vi "UT_FX5U_SLMP.vi"() -> ()   [LabVIEW 2019]
uses:
  FX5U SLMP Binary/FX5U SLMP Binary.lvlib
panel:
  in  "IP:Port":string="192.168.3.70:1234"
  out "Success":bool
  out "Error":bool
  in  "Close API":bool
  out "TCP connected":bool
  in  "D Array":i16[](array[numeric])=[0, -30, 0, 50, 79, 69, 90, 0, 0, 80, 0, 0]
  in  "Wr D Length (U16)":u16=10
  in  "Wr D Position (U32)":u32=7500
  in  "Write Multi-D":bool
  in  "Wr M Length (U16)":u16=10
  in  "Wr M Start Position (U32)":u32=6500
  in  "M Data input":bool[](array[boolean])=[FALSE, FALSE, TRUE, FALSE, FALSE, TRUE, FALSE, FALSE, FALSE, TRUE, FALSE, FALSE, FALSE, FALSE, TRUE, TRUE]
  in  "Write Multi-M":bool
  in  "Rd D Length (U16)":u16=12
  in  "Rd D Start Position (U32)":u32=7500
  in  "Write Unit-D":bool
  in  "Read Multi-D":bool
  out "Error Out":errorcluster
  in  "Error In":errorcluster
  out "D Data out":i16[](array[numeric])=[0, 0, -12288, 0, -1, 3, 2, 0, 208, -256, 1023, 6656]
  out "M  Data out":bool[](array[boolean])=[FALSE, FALSE, FALSE, FALSE, FALSE, FALSE, FALSE, FALSE, FALSE, FALSE, FALSE, FALSE, FALSE, FALSE, TRUE, FALSE, FALSE, TRUE, FALSE, FALSE]
  in  "Wr D Position (U32)":u32=7500
  in  "D Data In":i16=50
  in  "M Data In":bool
  in  "Wr M Position (U32)":u32
  in  "Rd M Length (U16)":u16=20
  in  "Rd M Start Position (U32)":u32=6500
  in  "stop":bool
  in  "Read Multi-M":bool
  in  "Write Unit-M":bool
  in  "Connect PLC":bool
  # "傳輸格式: BINARY\n參考FX5U SLMP手冊編輯通訊架構\n已測試: FX5U 64M型號"
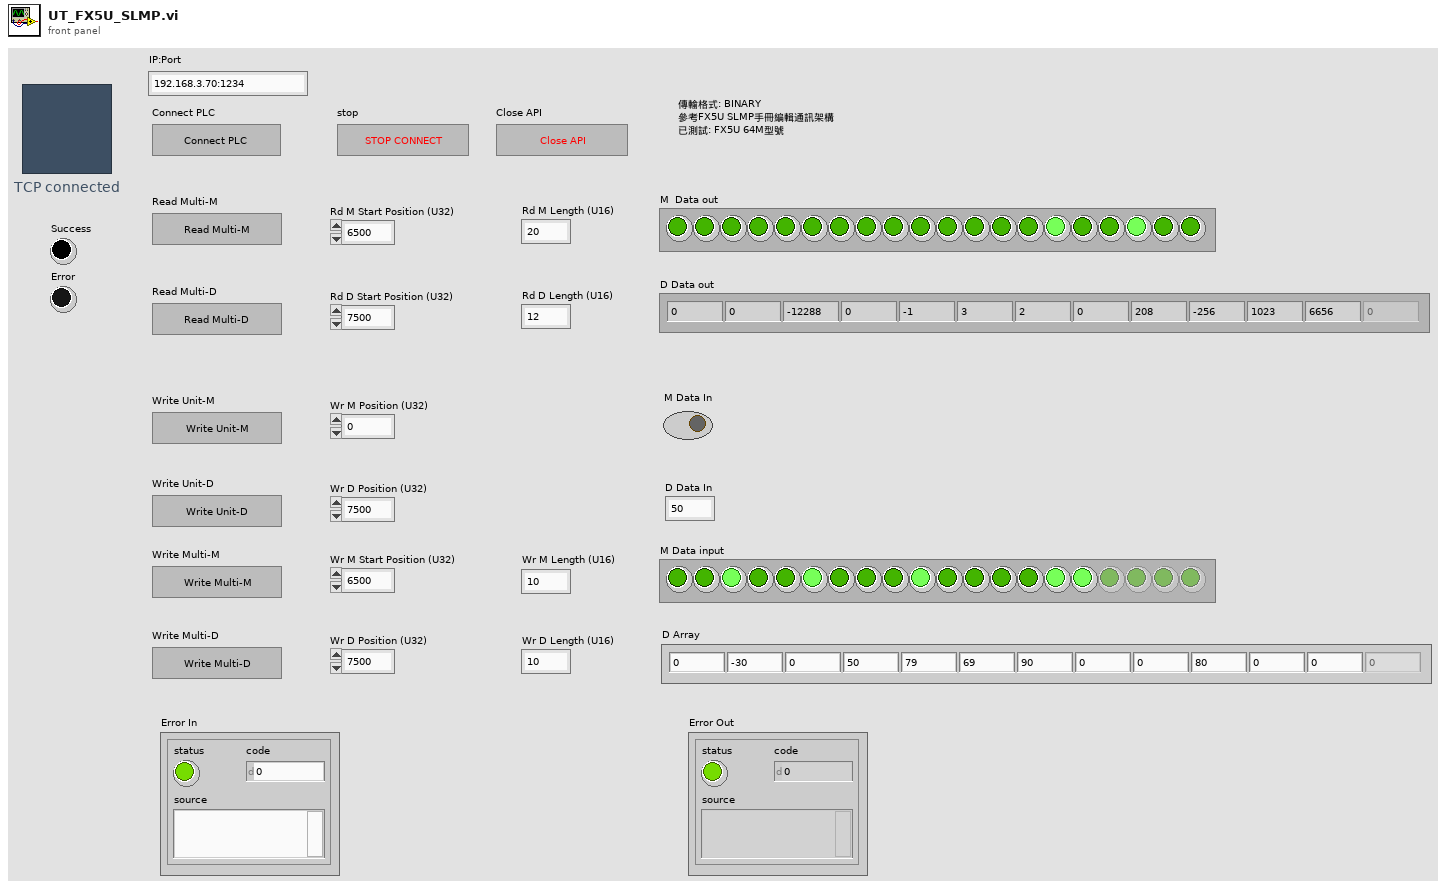
[diagram p1: front panel]
types:
  T1 = typedef "FX5U SLMP Binary.lvlib/Data Cluster.ctl" = cluster{"M Array":bool[], "D Array":i16[]}
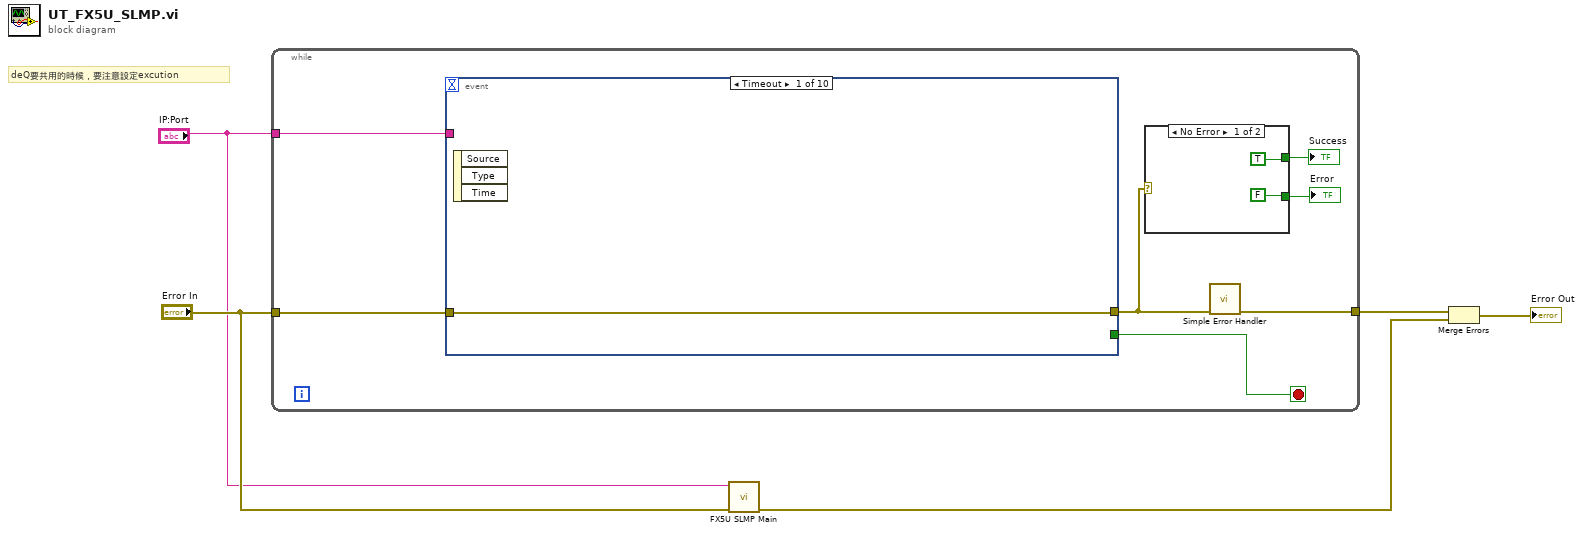
[diagram p0: block diagram]
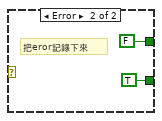
[diagram p2: hidden frame]
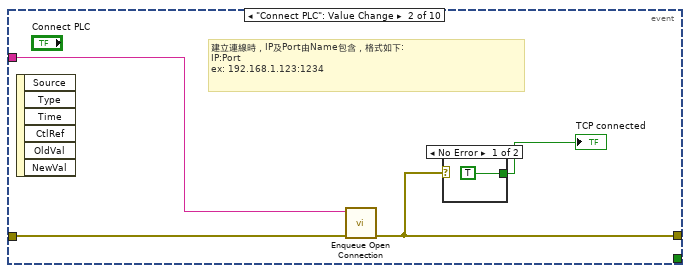
[diagram p3: hidden frame]
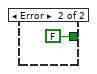
[diagram p4: hidden frame]
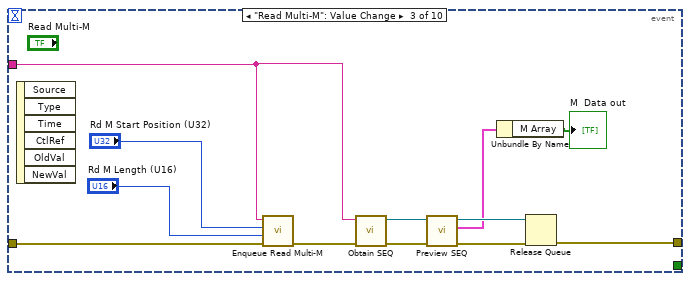
[diagram p5: hidden frame]
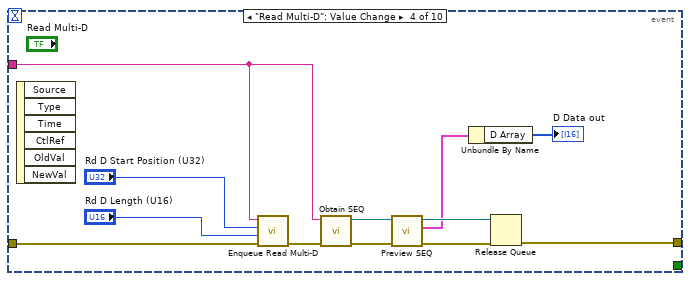
[diagram p6: hidden frame]
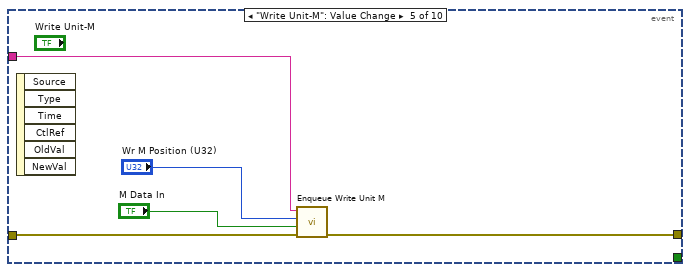
[diagram p7: hidden frame]
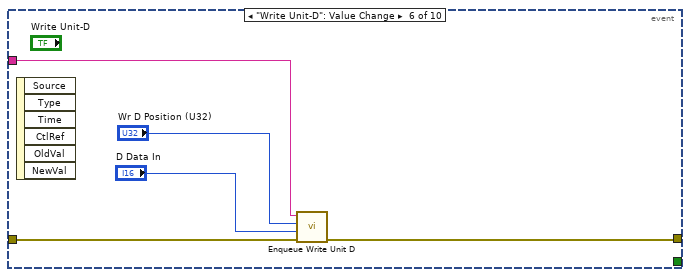
[diagram p8: hidden frame]
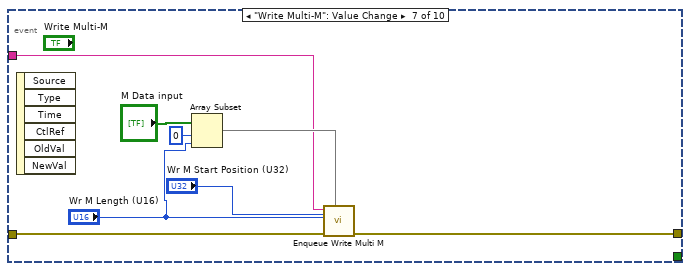
[diagram p9: hidden frame]
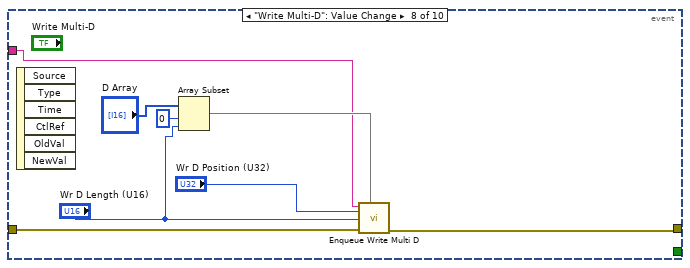
[diagram p10: hidden frame]
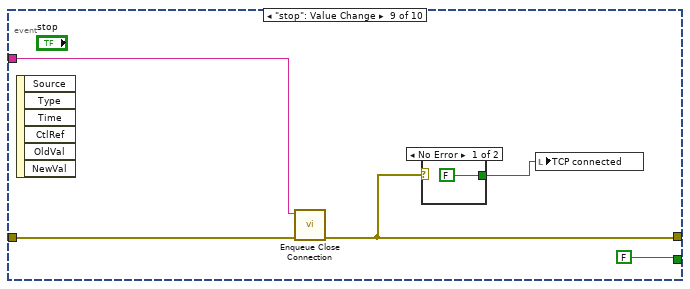
[diagram p11: hidden frame]
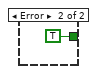
[diagram p12: hidden frame]
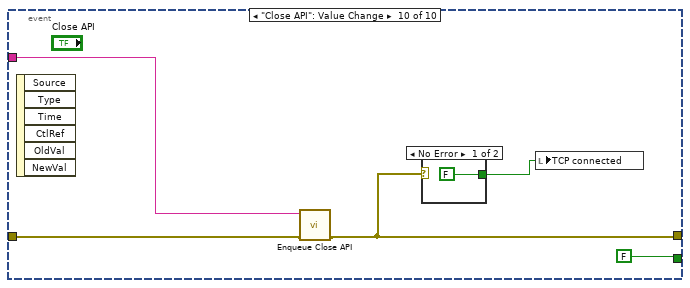
[diagram p13: hidden frame]
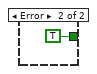
[diagram p14: hidden frame]
diagram:
  # "deQ要共用的時候，要注意設定excution"
  n1 = while {
    tunnel: "Error In" -> [w12]
    tunnel: [w11] -> w5
    tunnel: "IP:Port" -> [w6]
    stop <- w10 stop-if-true
    n2 = event shown="[0] Timeout" {
      selector: _ -> [_ _ _ _ _ _ _ _ _ _]
      dyn-events: _ -> [_ _ _ _ _ _ _ _ _ _]
      timeout: _ -> [_ _ _ _ _ _ _ _ _ _]
      tunnel: w12 -> [w17 w21 w35 w39 w50 w57 w64 w73 w78 w83]
      tunnel: [w17 w20 w31 w43 w49 w56 w63 w72 w76 w82] -> w7
      tunnel: [_ _ _ _ _ _ _ _ FALSE FALSE] -> w10
      tunnel: w6 -> [_ w18 w24 w36 w48 w53 w58 w66 w74 w81]
      event Timeout {
        n3 = event-data() -> ()  [unwired: 1 in, 3 out]
      }
      event "Connect PLC": Value Change {
        # "建立連線時，IP及Port由Name包含，格式如下:\nIP:Port\nex: 192.168.1.123:1234"
        n4 = event-data() -> ()  [unwired: 1 in, 6 out]
        n5 = call "Enqueue Open Connection.vi"("Error In"=w21, "Name"=w18) -> ("Error Out"=w20:errorcluster)  [unwired: 9 in]
        n6 = case shown="No Error" w20 {
          tunnel: [TRUE ("TCP connected") FALSE ("TCP connected")] -> w19
          frame No Error {
          }
          frame Error {
          }
        }
        "TCP connected" <- w19
      }
      event "Read Multi-M": Value Change {
        n7 = event-data() -> ()  [unwired: 1 in, 6 out]
        n8 = call "Enqueue Read Multi-M.vi"("Error In"=w35, "Length (U16)"="Rd M Length (U16)", "Start Position (U32)"="Rd M Start Position (U32)", "Name"=w24) -> ("Error Out"=w32:errorcluster)  [unwired: 7 in]
        n9 = call "Obtain SEQ.vi"("Error In"=w32, "Name"=w24) -> ("Error Out"=w30:errorcluster, "SEQ out"=w28:refnum<queue>)  [unwired: 8 in]
        n10 = call "Preview SEQ.vi"("Error In"=w30, "SEQ in"=w28) -> ("Error Out"=w29:errorcluster, "Data Cluster"=w26:T1, "SEQ out"=w27:refnum<queue>)  [unwired: 7 in]
        n11 = Unbundle By Name(w26) -> ("M Array"=→"M  Data out":bool[])
        n12 = Release Queue(queue=w27, error in (no error)=w29) -> (error out=w31:errorcluster)  [unwired: 1 in, 2 out]
      }
      event "Read Multi-D": Value Change {
        n13 = event-data() -> ()  [unwired: 1 in, 6 out]
        n14 = call "Enqueue Read Multi-D.vi"("Error In"=w39, "Length (U16)"="Rd D Length (U16)", "Start Position (U32)"="Rd D Start Position (U32)", "Name"=w36) -> ("Error Out"=w42:errorcluster)  [unwired: 7 in]
        n15 = call "Obtain SEQ.vi"("Error In"=w42, "Name"=w36) -> ("Error Out"=w47:errorcluster, "SEQ out"=w45:refnum<queue>)  [unwired: 8 in]
        n16 = call "Preview SEQ.vi"("Error In"=w47, "SEQ in"=w45) -> ("Error Out"=w46:errorcluster, "Data Cluster"=w38:T1, "SEQ out"=w44:refnum<queue>)  [unwired: 7 in]
        n17 = Unbundle By Name(w38) -> ("D Array"=→"D Data out":i16[])
        n18 = Release Queue(queue=w44, error in (no error)=w46) -> (error out=w43:errorcluster)  [unwired: 1 in, 2 out]
      }
      event "Write Unit-M": Value Change {
        n19 = event-data() -> ()  [unwired: 1 in, 6 out]
        n20 = call "Enqueue Write Unit M.vi"("Error In"=w50, "Data In"="M Data In", "Position (U32)"="Wr M Position (U32)", "Name"=w48) -> ("Error Out"=w49:errorcluster)  [unwired: 7 in]
      }
      event "Write Unit-D": Value Change {
        n21 = event-data() -> ()  [unwired: 1 in, 6 out]
        n22 = call "Enqueue Write Unit D.vi"("Error In"=w57, "D Data In"="D Data In", "Position (U32)"="Wr D Position (U32)", "Name"=w53) -> ("Error Out"=w56:errorcluster)  [unwired: 7 in]
      }
      event "Write Multi-M": Value Change {
        n23 = event-data() -> ()  [unwired: 1 in, 6 out]
        n24 = Array Subset(array="M Data input", index=0, length="Wr M Length (U16)") -> (w59:bool[])
        n25 = call "Enqueue Write Multi M.vi"("Array"=w59, "Error In"=w64, "Length (U16)"="Wr M Length (U16)", "Position (U32)"="Wr M Start Position (U32)", "Name"=w58) -> ("Error Out"=w63:errorcluster)  [unwired: 6 in]
      }
      event "Write Multi-D": Value Change {
        n26 = event-data() -> ()  [unwired: 1 in, 6 out]
        n27 = Array Subset(array="D Array", index=0, length="Wr D Length (U16)") -> (w67:i16[])
        n28 = call "Enqueue Write Multi D.vi"("D Array"=w67, "Error In"=w73, "Length (U16)"="Wr D Length (U16)", "Position (U32)"="Wr D Position (U32)", "Name"=w66) -> ("Error Out"=w72:errorcluster)  [unwired: 6 in]
      }
      event "stop": Value Change {
        n29 = event-data() -> ()  [unwired: 1 in, 6 out]
        n30 = call "Enqueue Close Connection.vi"("Error In"=w78, "Name"=w74) -> ("Error Out"=w76:errorcluster)  [unwired: 9 in]
        n31 = case shown="No Error" w76 {
          tunnel: [FALSE ("TCP connected") TRUE ("TCP connected")] -> w75
          frame No Error {
          }
          frame Error {
          }
        }
        n32 = local write "TCP connected"(w75) -> ()
      }
      event "Close API": Value Change {
        n33 = event-data() -> ()  [unwired: 1 in, 6 out]
        n34 = call "Enqueue Close API.vi"("Error In"=w83, "Name"=w81) -> ("Error Out"=w82:errorcluster)  [unwired: 9 in]
        n35 = case shown="No Error" w82 {
          tunnel: [FALSE ("TCP connected") TRUE ("TCP connected")] -> w84
          frame No Error {
          }
          frame Error {
          }
        }
        n36 = local write "TCP connected"(w84) -> ()
      }
    }
    n37 = case shown="No Error" w7 {
      tunnel: [TRUE FALSE] -> w9
      tunnel: [FALSE TRUE] -> w8
      frame No Error {
      }
      frame Error {
        # "把eror記錄下來"
      }
    }
    "Error" <- w8
    "Success" <- w9
    n38 = call <vilib>:"Simple Error Handler.vi"("error in (no error)"=w7) -> ("error out"=w11:errorcluster)  [unwired: 4 in, 4 out]
  }
  n39 = call "FX5U SLMP Main.vi"("Error In"="Error In", "Name"="IP:Port") -> ("Error Out"=w3:errorcluster)  [unwired: 9 in]
  n40 = Merge Errors(w5, w3) -> (→"Error Out":errorcluster)
